vi "Set Number Of Steps.vi"(10 "Number Of Steps":i32, 11 "Move Steps Command in":refnum<class "Move Steps Command.lvclass">) -> (3 "Move Steps Command out":refnum<class "Move Steps Command.lvclass">)   [LabVIEW 2016, in "Move Steps Command.lvclass"]
uses:
  Move Steps Command.lvclass
  Move Steps Command.lvclass/Move Steps Command.ctl
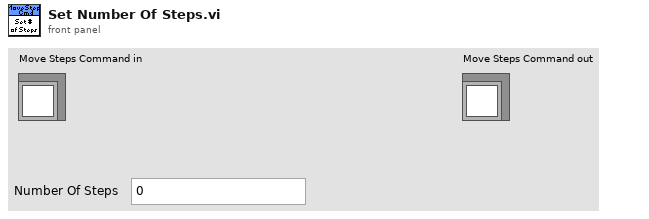
[diagram p1: front panel]
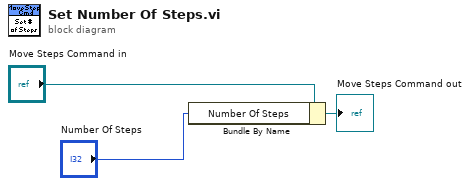
[diagram p0: block diagram]
diagram:
  n1 = Bundle By Name(cluster="Move Steps Command in", "Number Of Steps"="Number Of Steps") -> (→"Move Steps Command out":refnum<class "Move Steps Command.lvclass">)
